vi "Write Browse button visible.vi"(5 "Browse button visible":bool, 9 "Path in":refnum<class "Path.lvclass">) -> (3 "Path out":refnum<class "Path.lvclass">)   [LabVIEW 2014, in "Path.lvclass"]
uses:
  Path.lvclass
  Path.lvclass/Path.ctl
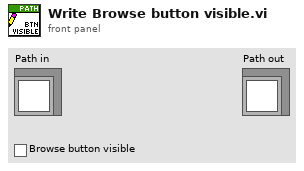
[diagram p1: front panel]
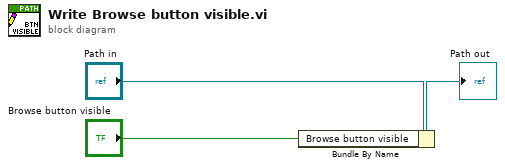
[diagram p0: block diagram]
diagram:
  n1 = Bundle By Name(cluster="Path in", "Browse button visible"="Browse button visible") -> (→"Path out":refnum<class "Path.lvclass">)
